vi "PC Recv Event.vi"(0 "RTsend/PCrecv CMD":T1, 2 "Mode":T2, 7 "Flattened Data":string, 11 "Error In":errorcluster) -> (4 "RTsend PCrecv Cluster":refnum<user-event>, 15 "Error Out":errorcluster)   [LabVIEW 2019]
uses:
  Event Mode.ctl
  RT/RTsend PCrecv CMD.ctl
  RT/RTsend PCrecv Cluster.ctl
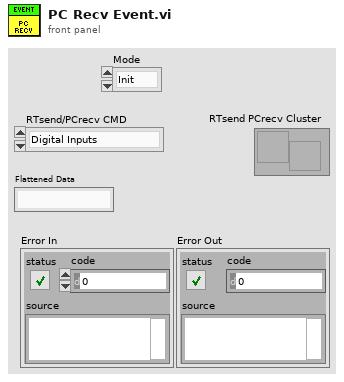
[diagram p1: front panel]
types:
  T1 = typedef "RTsend PCrecv CMD.ctl" = enum16{"Digital Inputs", "Connected?", "Data", "Data 2", "Cal2PC"}
  T2 = typedef "Event Mode.ctl" = enum16{"Init", "Get", "Set", "Destroy"}
  T3 = typedef "RTsend PCrecv Cluster.ctl" = cluster{"RTsend/PCrecv CMD":T1, "Flattened Data":string}
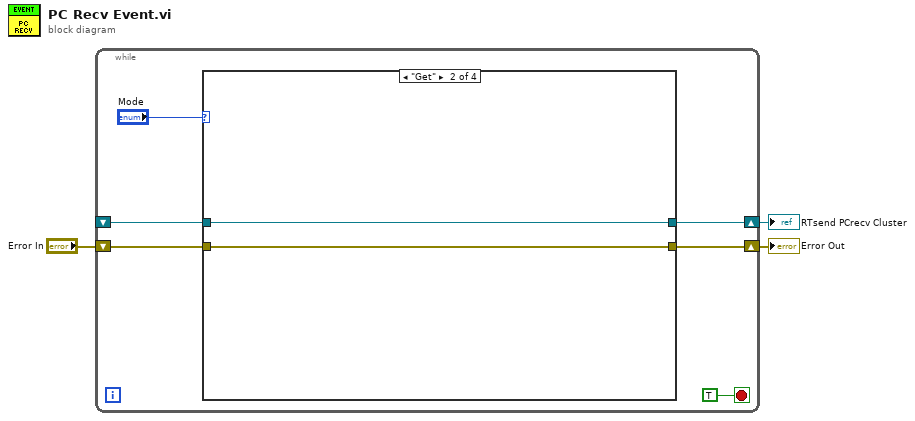
[diagram p0: block diagram]
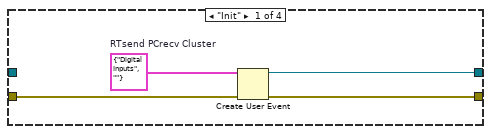
[diagram p2: hidden frame]
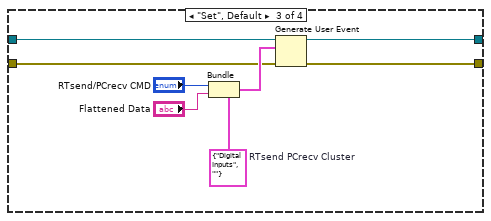
[diagram p3: hidden frame]
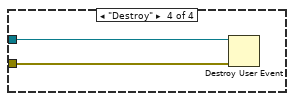
[diagram p4: hidden frame]
diagram:
  n1 = while {
    shift-right: [w5] -> w1
    shift-left: _ -> [w4]
    shift-right: [w7] -> w2
    shift-left: "Error In" -> [w6]
    stop <- TRUE stop-if-true
    n2 = case shown="\"Get\"" "Mode" {
      tunnel: [w13 w15 w20 _] -> w7
      tunnel: w6 -> [w12 w15 w21 w25]
      tunnel: [w10 w14 w16 _] -> w5
      tunnel: w4 -> [_ w14 w17 w24]
      frame "Init" {
        w11 = T3 {"RTsend/PCrecv CMD"=enum."Digital Inputs", "Flattened Data"=""}  # RTsend PCrecv Cluster
        n3 = Create User Event(user event datatype=w11, error in=w12) -> (user event=w10:refnum<user-event>, error out=w13:errorcluster)
      }
      frame "Get" {
      }
      frame "Set", Default {
        w19 = T3 {"RTsend/PCrecv CMD"=enum."Digital Inputs", "Flattened Data"=""}  # RTsend PCrecv Cluster
        n4 = Bundle(cluster=w19, "RTsend/PCrecv CMD"="RTsend/PCrecv CMD", "Flattened Data"="Flattened Data") -> (w22:T3)
        n5 = Generate User Event(user event=w17, event data cluster=w22, error in=w21) -> (user event out=w16:refnum<user-event>, error out=w20:errorcluster)  [unwired: 1 in]
      }
      frame "Destroy" {
        n6 = Destroy User Event(user event=w24, error in=w25) -> ()  [unwired: 1 out]
      }
    }
  }
  "Error Out" <- w2
  "RTsend PCrecv Cluster" <- w1
